vi "iscorner.vi"(8 "index2":dbl, 9 "index1":dbl, 11 "intensity values":dbl[][](array[numeric])) -> (0 "isCorner":bool)   [LabVIEW 2016]
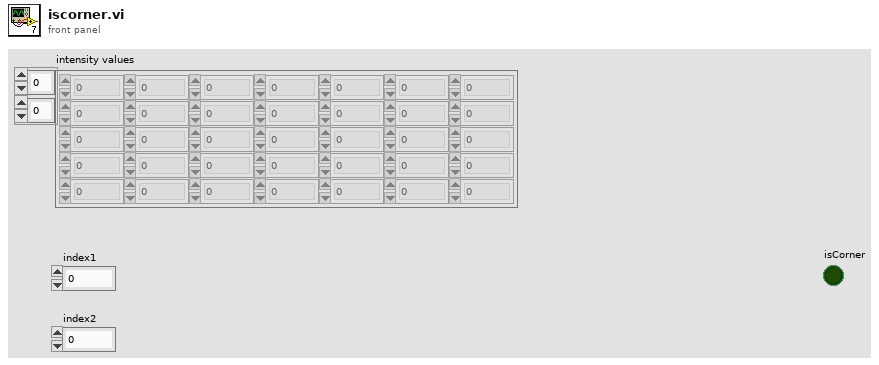
[diagram p1: front panel]
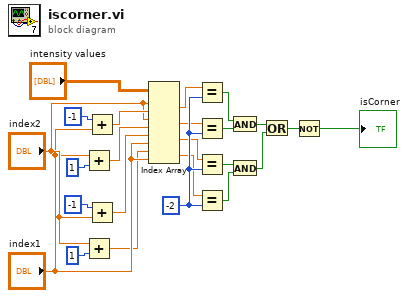
[diagram p0: block diagram]
diagram:
  w18 = -2
  n1 = Add(x="index1", y=1) -> (x+y=w6:dbl)
  n2 = Add(x="index2", y=1) -> (x+y=w2:dbl)
  n3 = Add(x=-1, y="index1") -> (x+y=w7:dbl)
  n4 = Add(x=-1, y="index2") -> (x+y=w3:dbl)
  n5 = Index Array(array="intensity values", index (row) #1="index2", index (col) #1=w7, index (row) #2="index2", index (col) #2=w6, index (row) #3=w3, index (col) #3="index1", index (row) #4=w2, index (col) #4="index1") -> (element #1=w19:dbl, element #2=w17:dbl, element #3=w16:dbl, element #4=w15:dbl)
  n6 = Equal?(x=w19, y=w18) -> (x = y?=w14:bool)
  n7 = Equal?(x=w17, y=w18) -> (x = y?=w13:bool)
  n8 = Equal?(x=w16, y=w18) -> (x = y?=w12:bool)
  n9 = Equal?(x=w15, y=w18) -> (x = y?=w11:bool)
  n10 = And(x=w14, y=w13) -> (x .and. y?=w10:bool)
  n11 = And(x=w12, y=w11) -> (x .and. y?=w9:bool)
  n12 = Or(x=w10, y=w9) -> (x .or. y?=w8:bool)
  n13 = Not(x=w8) -> (.not. x?=→"isCorner":bool)
